vi "vi.vi"() -> ()   [LabVIEW 2019]
uses:
  <vilib>/Instr/_visa.llb/VISA Configure Serial Port (Instr).vi
panel:
  in  "write buffer":string
  out "return count 2":u32
  out "return count":u32
  in  "milliseconds to wait":u32
  out "read buffer":string
  in  "byte count":u32
  in  "VISA resource name":refnum<visa-resource-name>
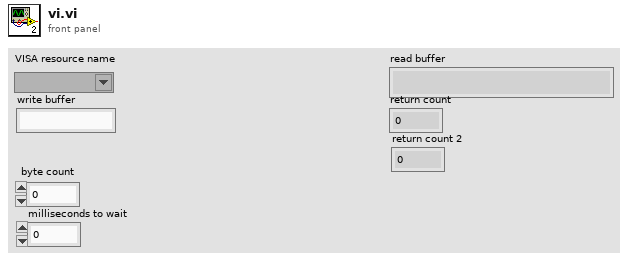
[diagram p1: front panel]
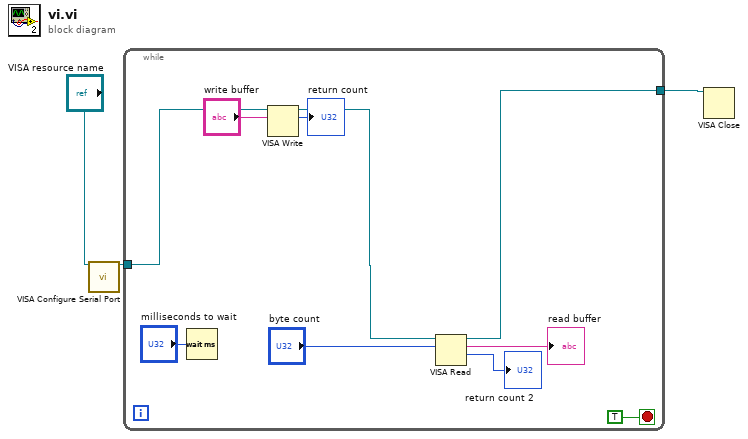
[diagram p0: block diagram]
diagram:
  n1 = call-poly "VISA Configure Serial Port"("VISA resource name"="VISA resource name") -> ("VISA resource name out"=w2:refnum<visa-resource-name>)  [unwired: 13 in, 1 out]
  n2 = while {
    tunnel: [w10] -> w3
    tunnel: w2 -> [w9]
    stop <- TRUE stop-if-true
    n3 = Wait (ms)(milliseconds to wait="milliseconds to wait") -> ()  [unwired: 1 out]
    n4 = VISA Write(VISA resource name=w9, write buffer="write buffer") -> (VISA resource name out=w5:refnum<visa-resource-name>, return count=→"return count":u32)  [unwired: 1 in, 1 out]
    n5 = VISA Read(VISA resource name=w5, byte count="byte count") -> (VISA resource name out=w10:refnum<visa-resource-name>, read buffer=→"read buffer":string, return count=→"return count 2":u32)  [unwired: 1 in, 1 out]
  }
  n6 = VISA Close(VISA resource name=w3) -> ()  [unwired: 1 in, 1 out]
